vi "Generate Date Time String.vi"() -> (2 "Date time string with milliseconds":string, 3 "Date time string":string)   [LabVIEW 2020, in "RTAF.lvlib"]
uses:
  RTAF.lvlib
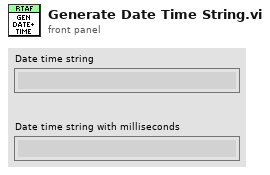
[diagram p1: front panel]
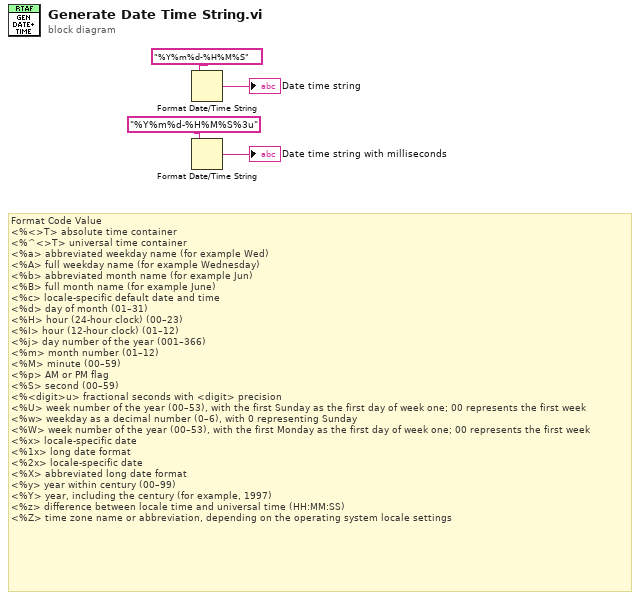
[diagram p0: block diagram]
diagram:
  # "Format Code Value \n<%<>T> absolute time container \n<%^<>T> universal time container \n<%a> abbreviated weekday name (for example Wed) \n<%A> full weekday name (for example Wednesday) \n<%b> abbreviated month name (for example Jun) \n<%B> full month name (for example June) \n<%c> locale-specific default date and time \n<%d> day of month (01–31) \n<%H> hour (24-hour clock) (00–23) \n<%I> hour (12-hour clock) (01–12) \n<%j> day number of the year (001–366) \n<%m> month number (01–12) \n<%M> minute (00–59) \n<%p> AM or PM flag \n<%S> second (00–59) \n<%<digit>u> fractional seconds with <digit> precision \n<%U> week number of the year (00–53), with the first Sunday as the first day of week one; 00 represents the first week \n<%w> weekday as a decimal number (0–6), with 0 representing Sunday \n<%W> week number of the year (00–53), with the first Monday as the first day of week one; 00 represents the first week \n<%x> locale-specific date \n<%1x> long date format \n<%2x> locale-specific date \n<%X> abbreviated long date format \n<%y> year within century (00–99) \n<%Y> year, including the century (for example, 1997) \n<%z> difference between locale time and universal time (HH:MM:SS) \n<%Z> time zone name or abbreviation, depending on the operating system locale settings"
  n1 = Format Date/Time String(time format string (%c)="%Y%m%d-%H%M%S") -> (date/time string=→"Date time string":string)  [unwired: 2 out]
  n2 = Format Date/Time String(time format string (%c)="%Y%m%d-%H%M%S%3u") -> (date/time string=→"Date time string with milliseconds":string)  [unwired: 2 out]
